vi "Move Syringe.vi"(8 "error in (no error)":errorcluster, 9 "Absolute Position (24000 steps)":u16=24000 max=48000 step=1, 10 "Address (1)":u16=1 max=15 step=1, 11 "VISA resource name":refnum<visa-resource-name>) -> (0 "error out":errorcluster, 1 "Busy":bool, 3 "VISA resource name out":refnum<visa-resource-name>)   [LabVIEW 2021, in "Copy of Kloehn V6 Series.lvlib"]
doc: "Moves the syringe to the position specified by the number. The range of positions allowed is dependent on the resolution of the instrument (12000, 24000, 48000)."
uses:
  Copy of Kloehn V6 Series.lvlib
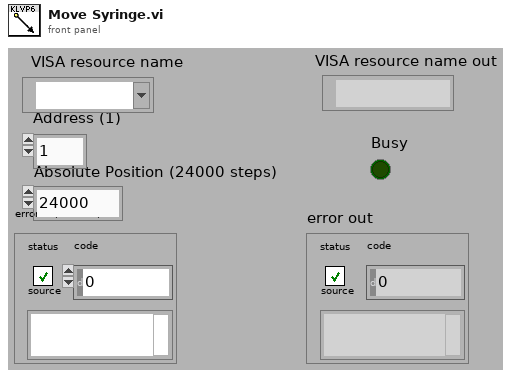
[diagram p1: front panel]
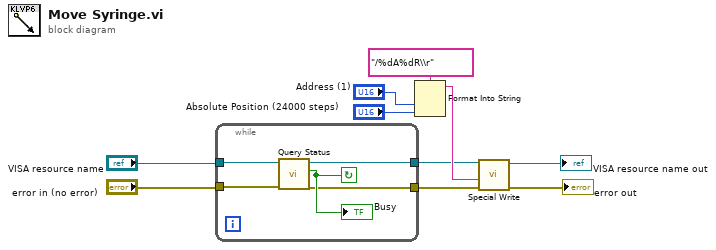
[diagram p0: block diagram]
diagram:
  n1 = while {
    tunnel: "VISA resource name" -> [w14]
    tunnel: [w13] -> w2
    tunnel: [w12] -> w1
    tunnel: "error in (no error)" -> [w11]
    stop <- w15 continue-if-true
    n2 = call "Query Status.vi"("error in (no error)"=w11, "VISA resource name"=w14) -> ("error out"=w12:errorcluster, "Status"=w15:bool, "VISA resource name out"=w13:refnum<visa-resource-name>)  [unwired: 7 in]
    "Busy" <- w15
  }
  n3 = Format Into String(format string="/%dA%dR\\r", "Address (1)", "Absolute Position (24000 steps)") -> (resulting string=w7:string)  [unwired: 2 in, 1 out]
  n4 = call "Special Write.vi"("error in (no error)"=w1, "Send String"=w7, "VISA resource name"=w2) -> ("error out"=→"error out":errorcluster, "VISA resource name out"=→"VISA resource name out":refnum<visa-resource-name>)  [unwired: 4 in, 3 out]
